vi "BPSK.vi"() -> ()   [LabVIEW 2014]
uses:
  <vilib>/Analysis/8numeric.llb/1D Numeric Integration.vi
  <vilib>/measure/NI_MABase.lvlib
  <vilib>/Analysis/NI_AALPro.lvlib
panel:
  out "Waveform Chart 3":i16[][](graph)
  out "Waveform Chart 2":i16[](graph)
  out "Waveform Chart":waveform(dbl)[](graph)
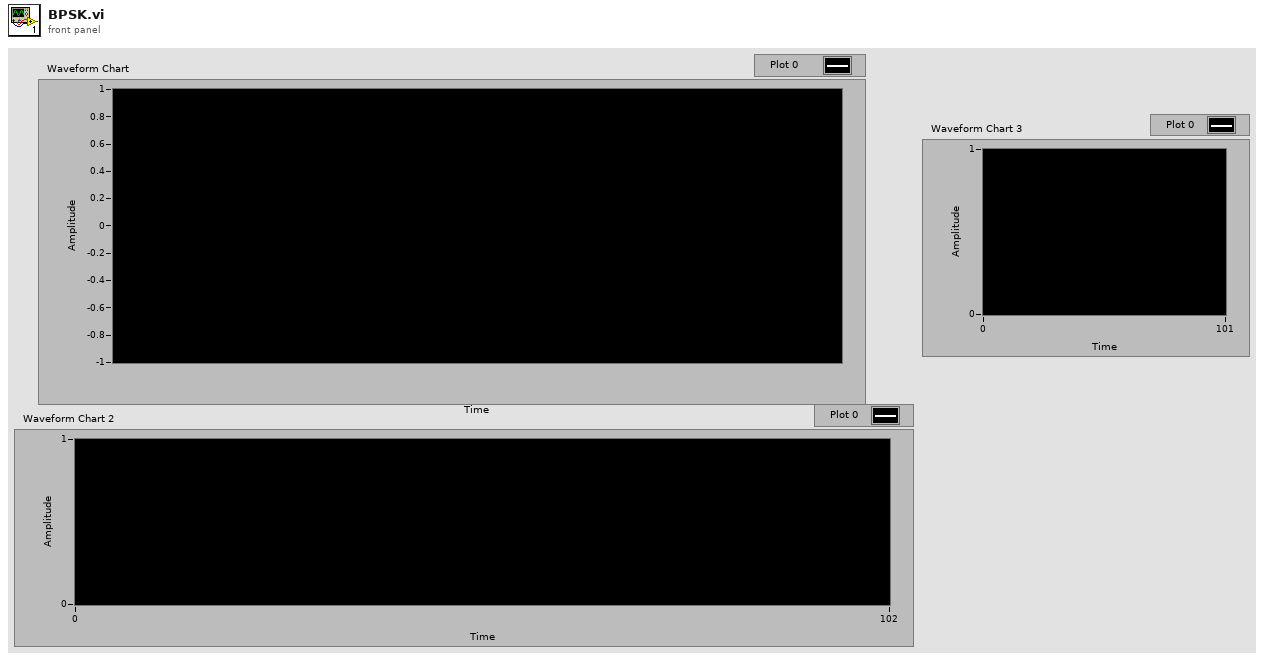
[diagram p1: front panel]
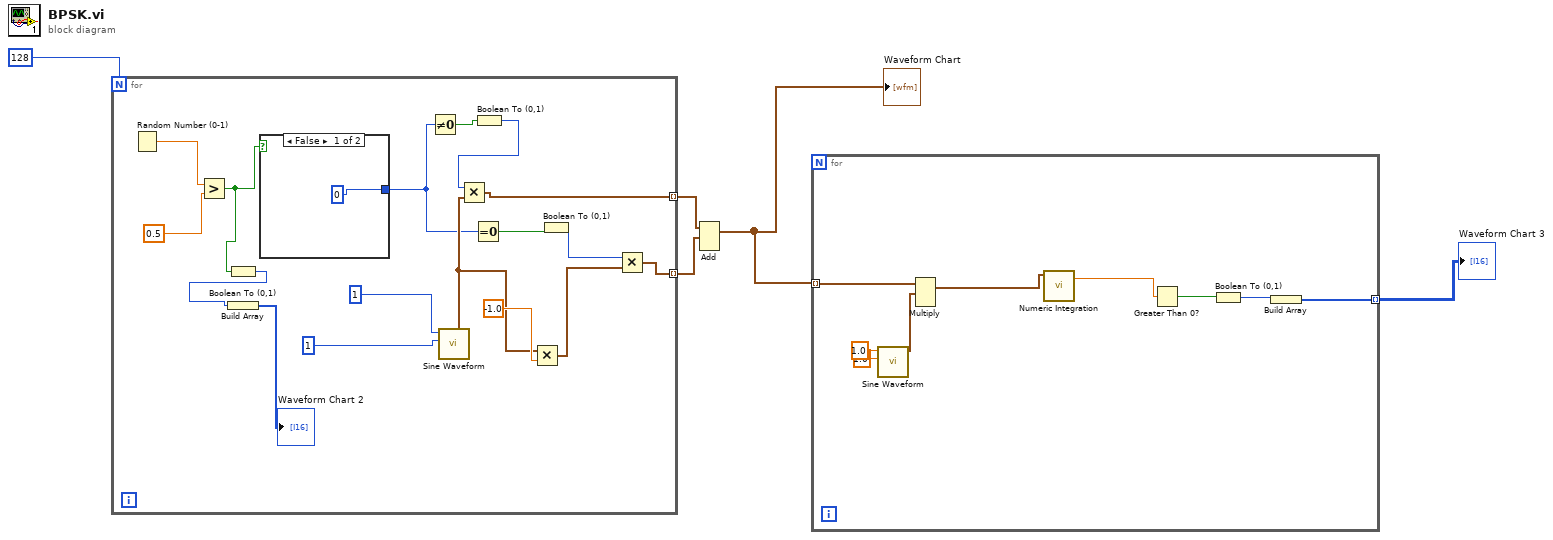
[diagram p0: block diagram]
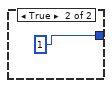
[diagram p2: hidden frame]
diagram:
  n1 = for {
    N: 128 ("Numeric") -> [_]
    tunnel: [w13] -> w4 mode=indexing
    tunnel: [w12] -> w3 mode=indexing
    n2 = Random Number (0-1)() -> (number: 0 to 1=w19:dbl)
    n3 = Greater?(x=w19, y=0.5) -> (0:w8:bool)
    n4 = Boolean To (0,1)(Boolean=w8) -> (0, 1=w7:i16)
    n5 = Build Array(w7) -> (→"Waveform Chart 2":i16[])
    n6 = case shown="False" w8 {
      tunnel: [0 1] -> w11
      frame False {
      }
      frame True {
      }
    }
    n7 = Not Equal To 0?(x=w11) -> (x != 0?=w21:bool)
    n8 = call <vilib>:"Sine Waveform.vi"("amplitude"=1, "frequency"=1) -> ("signal out"=w16:waveform(dbl))  [unwired: 8 in, 1 out]
    n9 = Equal To 0?(x=w11) -> (x = 0?=w17:bool)
    n10 = Boolean To (0,1)(Boolean=w21) -> (0, 1=w22:i16)
    n11 = Multiply(x=w22, y=w16) -> (x*y=w13:waveform(dbl))
    n12 = Multiply(x=w16, y=-1.0) -> (x*y=w15:waveform(dbl))
    n13 = Boolean To (0,1)(Boolean=w17) -> (0, 1=w14:i16)
    n14 = Multiply(x=w14, y=w15) -> (x*y=w12:waveform(dbl))
  }
  n15 = Add(1:w3, 2:w4) -> (0:w2:waveform(dbl)[])  [unwired: 1 in, 1 out]
  "Waveform Chart" <- w2
  n16 = for {
    tunnel: w2 -> [w33] mode=indexing
    tunnel: [w25] -> w1 mode=indexing
    n17 = call <vilib>:"Sine Waveform.vi"("amplitude"=1.0, "frequency"=1.0) -> ("signal out"=w30:waveform(dbl))  [unwired: 8 in, 1 out]
    n18 = Multiply(1:w30, 2:w33) -> (0:w29:waveform(dbl))  [unwired: 1 in, 1 out]
    n19 = call-poly <vilib>:"Numeric Integration.vi"("Input Array"=w29) -> ("result"=w28:dbl)  [unwired: 2 in, 1 out]
    n20 = Greater Than 0?(x=w28) -> (x > 0?=w27:bool)
    n21 = Boolean To (0,1)(Boolean=w27) -> (0, 1=w26:i16)
    n22 = Build Array(w26) -> (w25:i16[])
  }
  "Waveform Chart 3" <- w1
